vi "build_packet.vi"(10 "universe":u16, 11 "Data In":u8[](array[numeric])) -> (3 "Packet Out":u8[](array[numeric]))   [LabVIEW 2023]
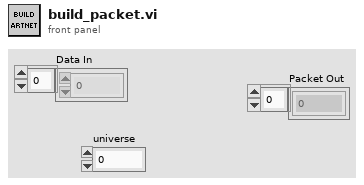
[diagram p1: front panel]
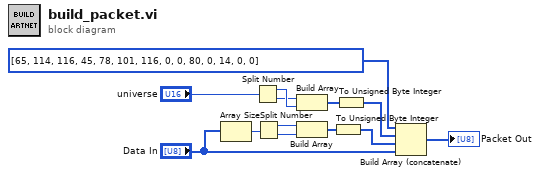
[diagram p0: block diagram]
diagram:
  n1 = Array Size(array="Data In") -> (size(s)=w7:i32)
  n2 = Split Number(x="universe") -> (hi(x)=w13:u8, lo(x)=w12:u8)
  n3 = Split Number(x=w7) -> (hi(x)=w6:u16, lo(x)=w5:u16)
  n4 = Build Array(w12, w13) -> (w9:u8[])
  n5 = Build Array(w6, w5) -> (w4:u16[])
  n6 = To Unsigned Byte Integer(number=w4) -> (unsigned 8bit integer=w3:u8[])
  n7 = To Unsigned Byte Integer(number=w9) -> (unsigned 8bit integer=w8:u8[])
  n8 = Build Array (concatenate)(u8[] [65, 114, 116, 45, 78, 101, 116, 0, 0, 80, 0, 14, 0, 0] ("Vorzeichenloses Byte-Array"), w8, w3, "Data In") -> (→"Packet Out":u8[])
